vi "Tek PS2520G Configure Supply24.vi"(0 "GPIB #":u8, 1 "voltage limit":dbl format="%.2f", 2 "Address":u8=8, 3 "channel (ch1:0)":u16(ring) items=["channel 1", "channel 2", "channel 3"], 4 "current limit":dbl format="%.3f", 5 "error in (no error)":errorcluster, 6 "Switch Output":bool, 7 "output (t:on)":bool=TRUE) -> (8 "error out":errorcluster)   [LabVIEW 2024]
panel:
  in  "ID query":bool
  in  "reset":bool
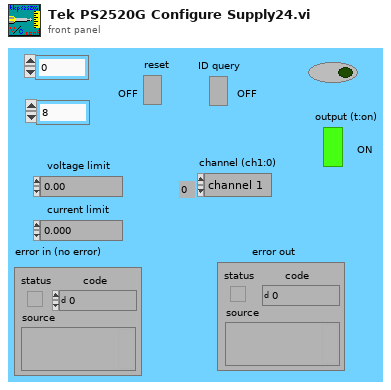
[diagram p1: front panel]
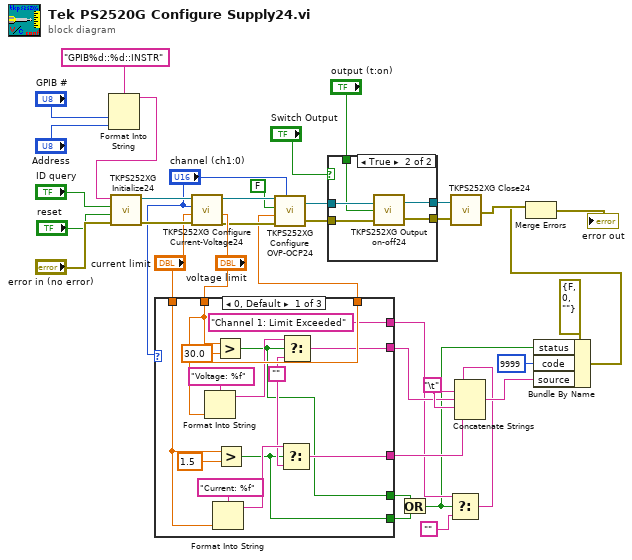
[diagram p0: block diagram]
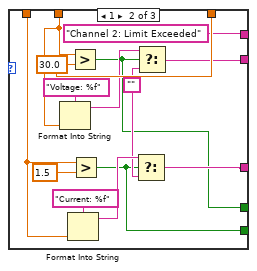
[diagram p3: hidden frame]
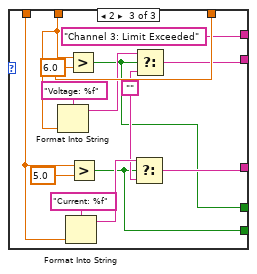
[diagram p4: hidden frame]
diagram:
  w24 = "\t"
  n1 = Format Into String(format string="GPIB%d::%d::INSTR" ("Format String"), "GPIB #", "Address") -> (resulting string=w12:string)  [unwired: 2 in, 1 out]
  n2 = call "TKPS252XG Initialize24.vi"("error in (no error)"="error in (no error)", "reset"="reset", "ID query"="ID query", "VISA session (for class)"=w12) -> ("error out"=w34:errorcluster, "VISA session"=w33:refnum<visa-resource-name>)
  n3 = case shown="0, Default" "channel (ch1:0)" {
    tunnel: "voltage limit" -> [w48 w58 w71]
    tunnel: "current limit" -> [w45 w54 w72]
    tunnel: ["Channel 1: Limit Exceeded" "Channel 2: Limit Exceeded" "Channel 3: Limit Exceeded"] -> w16
    tunnel: [w41 w56 w69] -> w23
    tunnel: [w40 w57 w68] -> w22
    tunnel: [w38 w53 w66] -> w18
    tunnel: [w39 w52 w67] -> w17
    tunnel: [w51 w65 w79] -> w1
    frame 0, Default {
      w43 = ""
      w51 = 30.0 ("y")
      n4 = Format Into String(format string="Voltage: %f" ("Format String"), w48) -> (resulting string=w47:string)  [unwired: 2 in, 1 out]
      n5 = Format Into String(format string="Current: %f" ("Format String"), w45) -> (resulting string=w44:string)  [unwired: 2 in, 1 out]
      n6 = Greater?(x=w48, y=w51) -> (0:w39:bool)
      n7 = Greater?(x=w45, y=1.5) -> (0:w38:bool)
      n8 = Select(t=w44, s=w38, f=w43) -> (s? t:f=w40:string)
      n9 = Select(t=w47, s=w39, f=w43) -> (s? t:f=w41:string)
    }
    frame 1 {
      w59 = ""
      w65 = 30.0 ("y")
      n10 = Format Into String(format string="Voltage: %f" ("Format String"), w58) -> (resulting string=w62:string)  [unwired: 2 in, 1 out]
      n11 = Format Into String(format string="Current: %f" ("Format String"), w54) -> (resulting string=w60:string)  [unwired: 2 in, 1 out]
      n12 = Greater?(x=w58, y=w65) -> (0:w52:bool)
      n13 = Greater?(x=w54, y=1.5) -> (0:w53:bool)
      n14 = Select(t=w60, s=w53, f=w59) -> (s? t:f=w57:string)
      n15 = Select(t=w62, s=w52, f=w59) -> (s? t:f=w56:string)
    }
    frame 2 {
      w73 = ""
      w79 = 6.0 ("y")
      n16 = Format Into String(format string="Voltage: %f" ("Format String"), w71) -> (resulting string=w76:string)  [unwired: 2 in, 1 out]
      n17 = Format Into String(format string="Current: %f" ("Format String"), w72) -> (resulting string=w74:string)  [unwired: 2 in, 1 out]
      n18 = Greater?(x=w71, y=w79) -> (0:w67:bool)
      n19 = Greater?(x=w72, y=5.0) -> (0:w66:bool)
      n20 = Select(t=w74, s=w66, f=w73) -> (s? t:f=w68:string)
      n21 = Select(t=w76, s=w67, f=w73) -> (s? t:f=w69:string)
    }
  }
  n22 = call "TKPS252XG Configure Current-Voltage24.vi"("voltage limit"="voltage limit", "error in (no error)"=w34, "current limit"="current limit", "channel (ch1:0)"="channel (ch1:0)", "VISA session"=w33) -> ("error out"=w7:errorcluster, "dup VISA session"=w6:refnum<visa-resource-name>)  [unwired: 1 in]
  n23 = call "TKPS252XG Configure OVP-OCP24.vi"("VISA session"=w6, "ocp (off:f)"=FALSE, "ovp limit"=w1, "error in (no error)"=w7, "channel (ch1:0)"="channel (ch1:0)") -> ("dup VISA session"=w10:refnum<visa-resource-name>, "error out"=w11:errorcluster)
  n24 = case shown="True" "Switch Output" {
    tunnel: w11 -> [w80 w86]
    tunnel: w10 -> [w81 w85]
    tunnel: [w80 w84] -> w9
    tunnel: [w81 w83] -> w8
    tunnel: "output (t:on)" -> [_ w82]
    frame False {
    }
    frame True {
      n25 = call "TKPS252XG Output on-off24.vi"("error in (no error)"=w86, "output (t:on)"=w82, "VISA session"=w85) -> ("error out"=w84:errorcluster, "dup VISA session"=w83:refnum<visa-resource-name>)
    }
  }
  n26 = Or(x=w17, y=w18) -> (x .or. y?=w13:bool)
  n27 = Select(t=w16, s=w13, f="") -> (s? t:f=w14:string)
  n28 = call "TKPS252XG Close24.vi"("error in (no error)"=w9, "VISA session"=w8) -> ("error out"=w28:errorcluster)
  n29 = Concatenate Strings(w14, w24, w23, w24, w22) -> (w21:string)
  n30 = Bundle By Name(cluster=errorcluster {"status"=FALSE, "code"=0, "source"=""} ("error out"), "status"=w13, "code"=9999, "source"=w21) -> (w27:errorcluster)
  n31 = Merge Errors(w28, w27) -> (→"error out":errorcluster)
